vi "GPIB Find all instruments sub.vi"() -> (0 "Array":cluster{"GPIB Addr":string, "*IDN":string}[](array[cluster]))   [LabVIEW 2012]
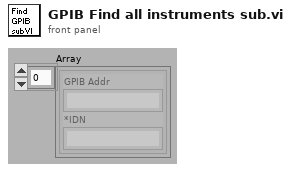
[diagram p1: front panel]
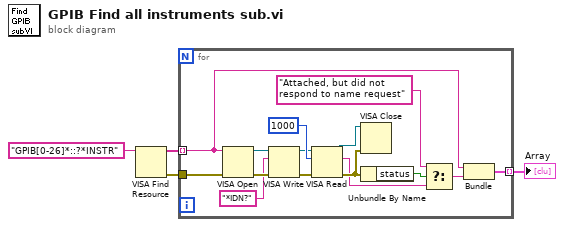
[diagram p0: block diagram]
diagram:
  n1 = VISA Find Resource(11:"GPIB[0-26]*::?*INSTR" ("expression (\"?*\")")) -> (0:w1:errorcluster, 3:w2:string[])  [unwired: 1 in, 2 out]
  n2 = for {
    tunnel: w2 -> [w11] mode=indexing
    tunnel: w1 -> [w17]
    tunnel: [w10] -> w4 mode=indexing
    n3 = VISA Open(error in (no error)=w17, VISA resource name=w11) -> (VISA resource name=w19:refnum<visa-resource-name>, error out=w18:errorcluster)  [unwired: 3 out]
    n4 = VISA Write(VISA resource name=w19, write buffer="*IDN?", error in (no error)=w18) -> (VISA resource name out=w13:refnum<visa-resource-name>, error out=w12:errorcluster)  [unwired: 1 out]
    n5 = VISA Read(VISA resource name=w13, byte count=u32 1000, error in (no error)=w12) -> (VISA resource name out=w14:refnum<visa-resource-name>, read buffer=w7:string, error out=w9:errorcluster)  [unwired: 1 out]
    n6 = VISA Close(VISA resource name=w14, error in (no error)=w9) -> ()  [unwired: 1 out]
    n7 = Unbundle By Name(w9) -> ("status"=w5:bool)
    n8 = Select(t="Attached, but did not respond to name request", s=w5, f=w7) -> (s? t:f=w6:string)
    n9 = Bundle(w11, "read buffer"=w6) -> (w10:cluster{string, "read buffer":string})  [unwired: 1 out]
  }
  "Array" <- w4
